vi "Tenney Process Data.vi"(0 "10 Minute Data Array Input":dbl[][](array[numeric]), 1 "Auto Control Input":bool, 5 "Tenney Environmental Chamber Data Input":T2, 11 "error in (no error)":errorcluster, 12 "Temperature Limits":T3={"Target Temperature Upper limit"=68.0, "Target Temperature Lower limit"=67.0, "Target Humidity Lower limit"=48.5, "Target Humidity Upper limit"=51.5, "Chamber Temperature Upper limit"=68.0, "Chamber Temperature Lower limit"=67.0, "Chamber Humidity Lower limit"=48.5, "Chamber Humidity Upper limit"=51.5, "Chamber Adjustment Increment (F)"=0.1, "Chamber Adjustment Interval (Minutes)"=10.0, "Chamber Adjustment Increment (%)"=0.1, "Chamber Adjustment Interval Fast (Minutes)"=5.0}, 13 "Viasala Data Output":T1) -> (3 "Elapsed Time (min)":dbl caption="Elapsed Time (s)", 4 "10 Minute Data Array Output":dbl[][](array[numeric]), 6 "Tenney Environmental Chamber Data Output":T2, 8 "Output CMD":string[](array[string]), 10 "Data CMD":dbl[](array[numeric]), 15 "error out":errorcluster)   [LabVIEW 2023]
uses:
  Drivers/Tidal Engineering/Type Definitions/Tenney Environmental Chamber Data.ctl
  controls/Tenney Temperature Limits.ctl
  Drivers/Viasala Indigo 520/Type Definitions/Viasala Indigo 520 Data.ctl
  <vilib>/Analysis/baseanly.llb/Mean (DBL).vi
  <vilib>/Analysis/NI_AALBase.lvlib
panel:
  out "Humidity Avg (%)":dbl format="%0.2f"
  out "Temp (Avg)":dbl format="%0.2f"
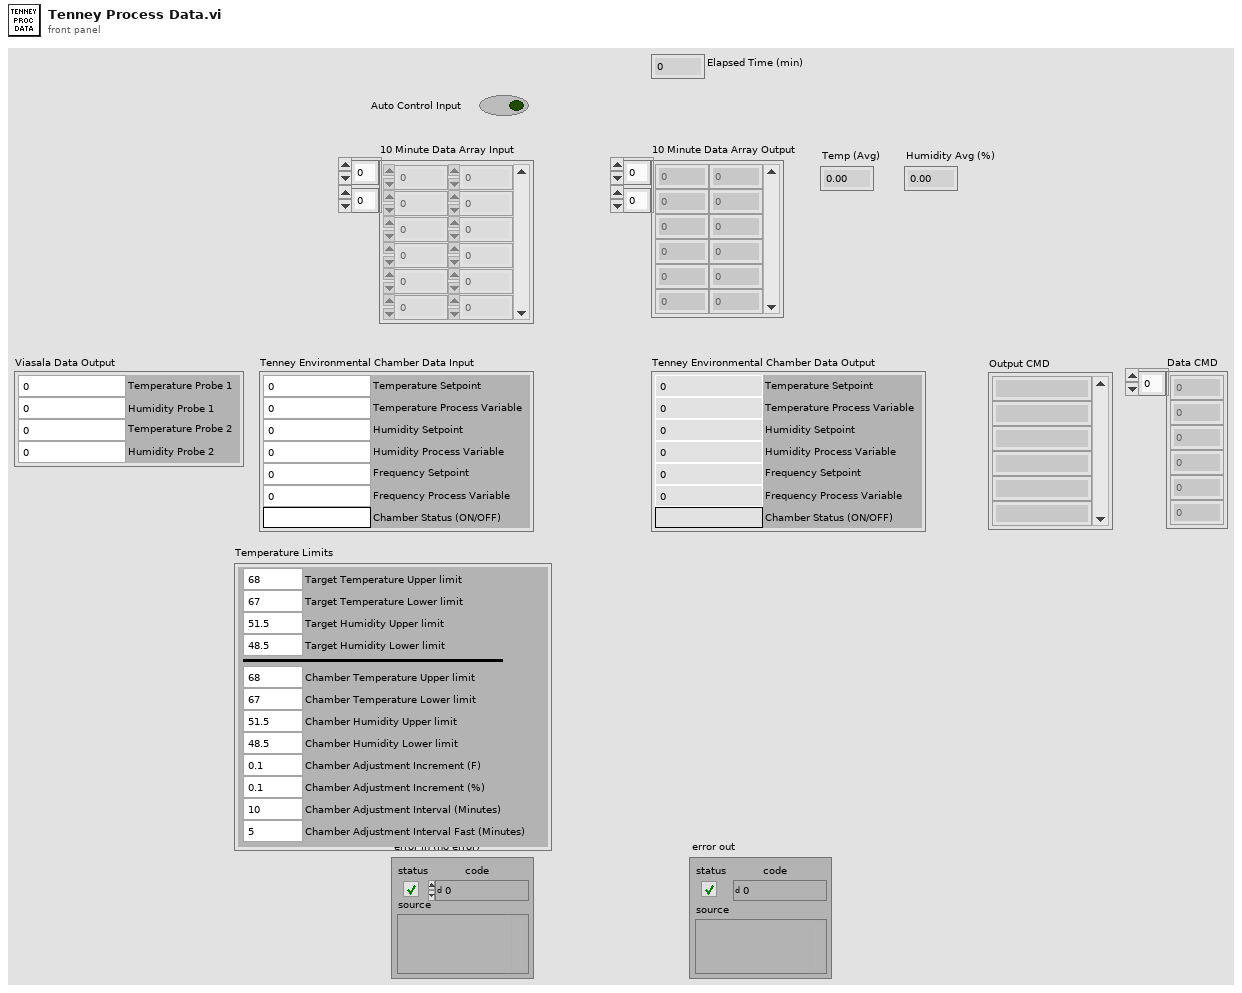
[diagram p1: front panel]
types:
  T1 = typedef "Viasala Indigo 520 Data.ctl" = cluster{"Temperature Probe 1":dbl, "Humidity Probe 1":dbl, "Temperature Probe 2":dbl, "Humidity Probe 2":dbl}
  T2 = typedef "Tenney Environmental Chamber Data.ctl" = cluster{"Temperature Setpoint":dbl, "Temperature Process Variable":dbl, "Humidity Setpoint":dbl, "Humidity Process Variable":dbl, "Frequency Setpoint":dbl, "Frequency Process Variable":dbl, "Chamber Status (ON/OFF)":string}
  T3 = typedef "Tenney Temperature Limits.ctl" = cluster{"Target Temperature Upper limit":dbl, "Target Temperature Lower limit":dbl, "Target Humidity Lower limit":dbl, "Target Humidity Upper limit":dbl, "Chamber Temperature Upper limit":dbl, "Chamber Temperature Lower limit":dbl, "Chamber Humidity Lower limit":dbl, "Chamber Humidity Upper limit":dbl, "Chamber Adjustment Increment (F)":dbl, "Chamber Adjustment Interval (Minutes)":dbl, "Chamber Adjustment Increment (%)":dbl, "Chamber Adjustment Interval Fast (Minutes)":dbl}
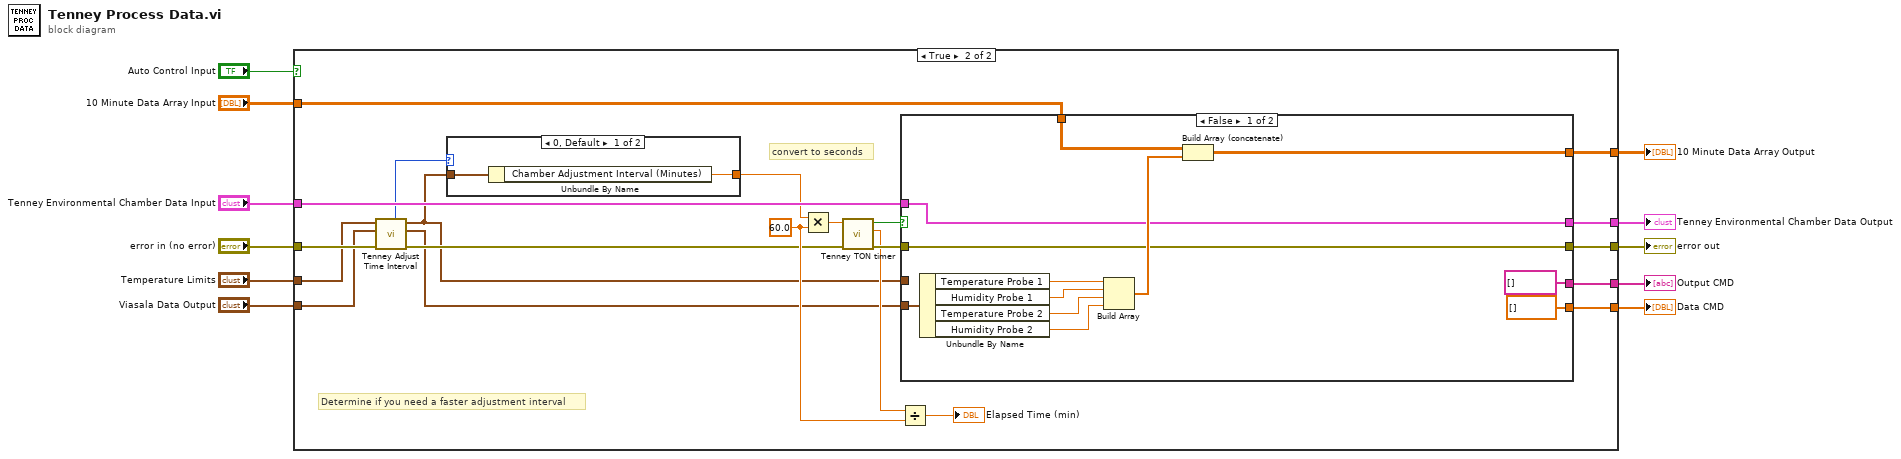
[diagram p0: block diagram]
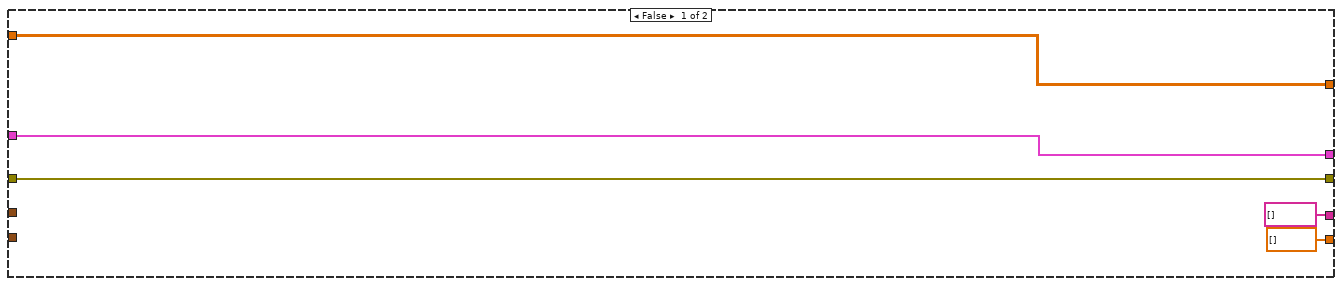
[diagram p2: hidden frame]
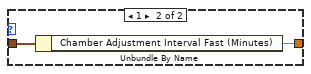
[diagram p3: hidden frame]
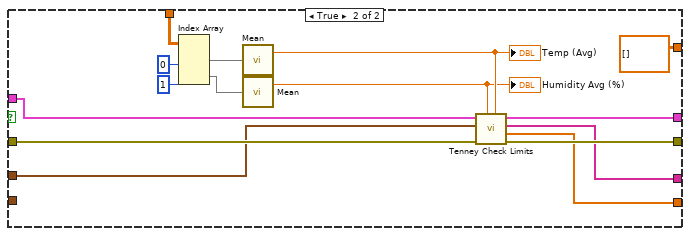
[diagram p4: hidden frame]
diagram:
  n1 = case shown="True" "Auto Control Input" {
    tunnel: "error in (no error)" -> [w16 w23]
    tunnel: "10 Minute Data Array Input" -> [w15 w35]
    tunnel: [w15 w34] -> w9
    tunnel: [w16 w33] -> w8
    tunnel: [string[] [] ("State CMD") w32] -> w7
    tunnel: "Tenney Environmental Chamber Data Input" -> [w14 w31]
    tunnel: [w14 w30] -> w4
    tunnel: [dbl[] [] ("Data CMD") w29] -> w3
    tunnel: "Viasala Data Output" -> [_ w21]
    tunnel: "Temperature Limits" -> [_ w20]
    frame False {
    }
    frame True {
      w25 = 60.0 ("y")
      # "Determine if you need a faster adjustment interval"
      # "convert to seconds"
      n2 = call "Tenney Adjust Time Interval.vi"("error in (no error)"=w23, "Viasala Data Input"=w21, "Temperature Limits Input"=w20) -> ("error out"=w22:errorcluster, "Viasala Data Output"=w19:T1, "Temperature Limits Output"=w18:T3, "Increment Selector (0-Normal or 1-Fast)"=w17:u8)  [unwired: 5 in]
      n3 = case shown="0, Default" w17 {
        tunnel: [w38 w41] -> w28
        tunnel: w18 -> [w39 w40]
        frame 0, Default {
          n4 = Unbundle By Name(w39) -> ("Chamber Adjustment Interval (Minutes)"=w38:dbl)
        }
        frame 1 {
          n5 = Unbundle By Name(w40) -> ("Chamber Adjustment Interval Fast (Minutes)"=w41:dbl)
        }
      }
      n6 = Multiply(x=w28, y=w25) -> (x*y=w27:dbl)
      n7 = call "Tenney TON timer.vi"("error in (no error)"=w22, "Time Target (s)"=w27) -> ("error out"=w37:errorcluster, "Elapsed Time (s)"=w26:dbl, "Time has Elapsed"=w36:bool)  [unwired: 7 in]
      n8 = Divide(x=w26, y=w25) -> (x/y=→"Elapsed Time (min)":dbl)
      n9 = case shown="False" w36 {
        tunnel: w37 -> [w48 w60]
        tunnel: w35 -> [w50 w68]
        tunnel: w31 -> [w47 w58]
        tunnel: [w49 dbl[][] []] -> w34
        tunnel: [w48 w59] -> w33
        tunnel: [string[] [] ("State CMD") w57] -> w32
        tunnel: [w47 w56] -> w30
        tunnel: [dbl[] [] ("Data CMD") w55] -> w29
        tunnel: w19 -> [w45 _]
        tunnel: w18 -> [_ w54]
        frame False {
          n10 = Unbundle By Name(w45) -> ("Temperature Probe 1"=w51:dbl, "Humidity Probe 1"=w52:dbl, "Temperature Probe 2"=w44:dbl, "Humidity Probe 2"=w43:dbl)
          n11 = Build Array(w51, w52, w44, w43) -> (w53:dbl[])
          n12 = Build Array (concatenate)(w50, w53) -> (w49:dbl[][])
        }
        frame True {
          n13 = Index Array(array=w68, index (col) #1=0 ("disabled index (col)"), index (col) #2=1 ("index (col)")) -> (element #1=w65:dbl[], element #2=w64:dbl[])  [unwired: 2 in]
          n14 = call-poly <vilib>:"Mean.vi"("X"=w65) -> ("mean"=w62:dbl)  [unwired: 1 out]
          "Temp (Avg)" <- w62
          n15 = call-poly <vilib>:"Mean.vi"("X"=w64) -> ("mean"=w61:dbl)  [unwired: 1 out]
          "Humidity Avg (%)" <- w61
          n16 = call "Tenney Check Limits.vi"("Temperature Average"=w62, "Humidity Average"=w61, "error in (no error)"=w60, "Temperature Limits"=w54, "Tenney Environmental Chamber Data Output in"=w58) -> ("error out"=w59:errorcluster, "Data CMD"=w55:dbl[], "State CMD"=w57:string[], "Tenney Environmental Chamber Data Output"=w56:T2)  [unwired: 3 in]
        }
      }
    }
  }
  "error out" <- w8
  "10 Minute Data Array Output" <- w9
  "Output CMD" <- w7
  "Tenney Environmental Chamber Data Output" <- w4
  "Data CMD" <- w3
